vi "SSL_set_connect_state.vi"(8 "error in (no error)":errorcluster, 11 "SSL-Lib in":refnum<class "SSL.lvclass">) -> (0 "error out":errorcluster, 3 "SSL-Lib out":refnum<class "SSL.lvclass">)   [LabVIEW 2013, in "OpenSSL Socket.lvlib" / "SSL.lvclass"]
uses:
  SSL.lvclass
  SSL-Lib/SSL-Lib.lvclass/SSL-Lib.ctl
  SSL.lvclass/SSL.ctl
  SSL-Lib/Read SSL Library Path.vi
  Read Handle.vi
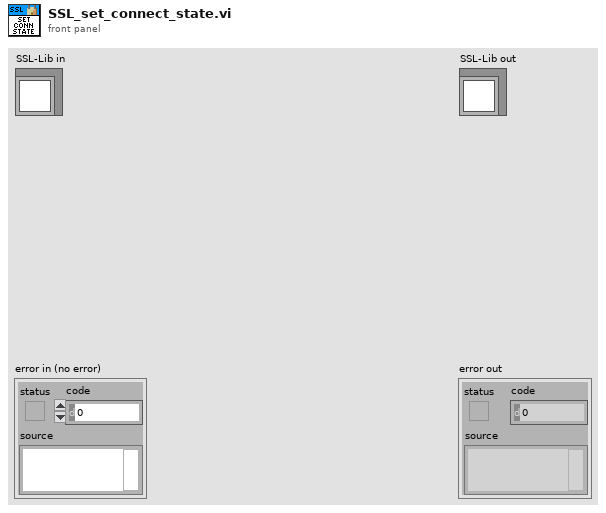
[diagram p1: front panel]
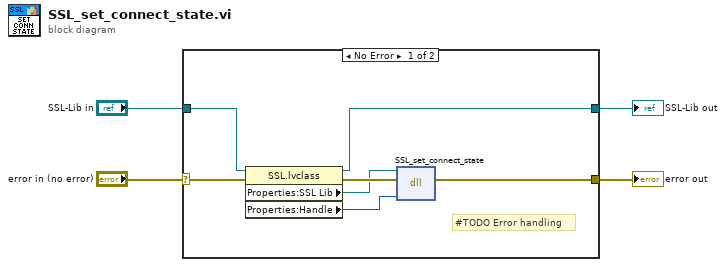
[diagram p0: block diagram]
diagram:
  n1 = case shown="No Error" "error in (no error)" {
    selector: "error in (no error)" -> [w11 w13]
    tunnel: [w10 w13] -> w3
    tunnel: [w9 w12] -> w1
    tunnel: "SSL-Lib in" -> [w8 w12]
    frame No Error {
      # "#TODO Error handling"
      n2 = property class="SSL.lvclass"(reference=w8, error in=w11) -> (reference out=w9:refnum<class "SSL.lvclass">, error out=w7:errorcluster, "Properties:SSL Lib"=w6:path, "Properties:Handle"=w5:u64)
      n3 = dll-call lib="C:/Program Files (x86)/National Instruments/Shared/nissl/NIssleay32.dll" fn="SSL_set_connect_state"(path in=w6, error in=w7, "SSL"=w5) -> (error out=w10:errorcluster)  [unwired: 3 in, 1 out]
    }
    frame Error {
    }
  }
  "error out" <- w3
  "SSL-Lib out" <- w1
